vi "Open Motors.vi"(3 "error in":errorcluster, 5 "Speed PID":T8={"P"=0.04995, "I"=4.995e-05, "D"=0.4995, "F Left"=0.05, "F Right"=0.05}) -> (0 "error out":errorcluster, 1 "Right Motor Refs":T1={"DeviceStatus"={"status"=FALSE, "code"=0, "source"=""}, "Type"=enum."PWM", "PWM"={"PWM Channel"=enum."PWM 1", "DeadBand"={"Name"="", "maxPositivePwm"=0, "minPositivePwm"=0, "centerPwm"=0, "maxNegativePwm"=0, "minNegativePwm"=0, "angularRange"=0}}, "CAN"={"Device Number"=0, "Control Mode"=enum."Percent VBus", "Semaphore"=refnum, "Max Vout"=12.0, "TalonSRX Control Mode"=enum."Percent VBus"}, "Invert"=FALSE}, 2 "Left Motor Refs":T1={"DeviceStatus"={"status"=FALSE, "code"=0, "source"=""}, "Type"=enum."PWM", "PWM"={"PWM Channel"=enum."PWM 1", "DeadBand"={"Name"="", "maxPositivePwm"=0, "minPositivePwm"=0, "centerPwm"=0, "maxNegativePwm"=0, "minNegativePwm"=0, "angularRange"=0}}, "CAN"={"Device Number"=0, "Control Mode"=enum."Percent VBus", "Semaphore"=refnum, "Max Vout"=12.0, "TalonSRX Control Mode"=enum."Percent VBus"}, "Invert"=FALSE})   [LabVIEW 2015]
uses:
  <vilib>/Rock Robotics/WPI/MotorControl/WPI_MotorControlDeviceRef.ctl
  <vilib>/Rock Robotics/WPI/MotorControl/WPI_MotorControlType.ctl
  <vilib>/Rock Robotics/SystemInterfaces/DIO/FPGA_DIOPWMChannel.ctl
  <vilib>/Rock Robotics/WPI/PWM/WPI_PWMDeadband.ctl
  <vilib>/Rock Robotics/WPI/CAN/Jaguar/SubVIs/WPI_CANJaguar_ControlMode.ctl
  <vilib>/Rock Robotics/WPI/CAN/TalonSRX/WPI_CANTalonSRX_APIControlMode.ctl
  <vilib>/Rock Robotics/WPI/CAN/TalonSRX/WPI_CANTalonSRX_APIFeedbackSelect.ctl
  <vilib>/Rock Robotics/WPI/CAN/TalonSRX/WPI_CANTalonSRX_BrakeOverride.ctl
  <vilib>/Rock Robotics/WPI/MotorControl/WPI_MotorControlOpenCANTalonSRX.vi
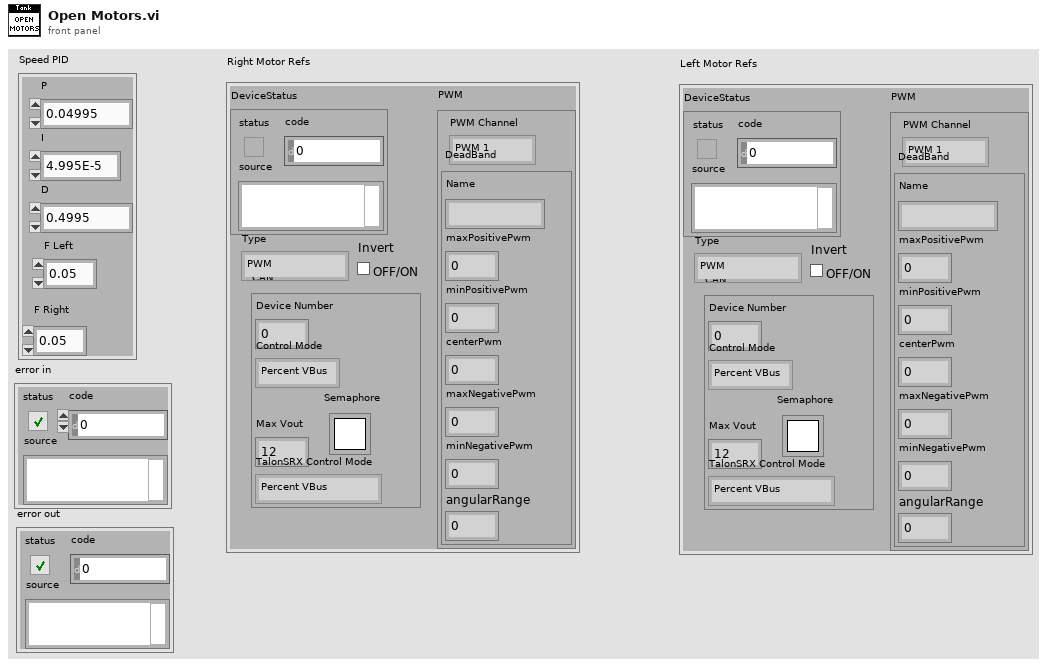
[diagram p1: front panel]
types:
  T1 = typedef "WPI_MotorControlDeviceRef.ctl" = cluster{"DeviceStatus":errorcluster, "Type":T2, "PWM":cluster{"PWM Channel":T3, "DeadBand":T4}, "CAN":cluster{"Device Number":u8, "Control Mode":T5, "Semaphore":T6, "Max Vout":dbl, "TalonSRX Control Mode":T7}, "Invert":bool}
  T2 = typedef "WPI_MotorControlType.ctl" = enum16{"PWM", "CAN", "CANTalonSRX"}
  T3 = typedef "FPGA_DIOPWMChannel.ctl" = enum8{"PWM 0", "PWM 1", "PWM 2", "PWM 3", "PWM 4", "PWM 5", "PWM 6", "PWM 7", "PWM 8", "PWM 9", "PWM MXP 0", "PWM MXP 1", "PWM MXP 2", "PWM MXP 3", "PWM MXP 4", "PWM MXP 5", "PWM MXP 6", "PWM MXP 7", "PWM MXP 8", "PWM MXP 9", "Invalid"}
  T4 = typedef "WPI_PWMDeadband.ctl" = cluster{"Name":string, "maxPositivePwm":i32, "minPositivePwm":i32, "centerPwm":i32, "maxNegativePwm":i32, "minNegativePwm":i32, "angularRange":u16}
  T5 = typedef "WPI_CANJaguar_ControlMode.ctl" = enum8{"Percent VBus", "Current", "Speed", "Position", "Voltage"}
  T6 = typedef "Semaphore RefNum" = refnum<k1>
  T7 = typedef "WPI_CANTalonSRX_APIControlMode.ctl" = enum8{"Percent VBus", "Speed", "Position", "Slave", "Unchanged / Invalid", "Voltage Compensation", "Current", "Motion Profile"}
  T8 = cluster{"P":dbl, "I":dbl, "D":dbl, "F Left":dbl, "F Right":dbl}
  T9 = typedef "WPI_CANTalonSRX_BrakeOverride.ctl" = enum8{"No Override", "Override to Coast", "Override to Brake"}
  T10 = typedef "WPI_CANTalonSRX_APIFeedbackSelect.ctl" = enum16{"Digital Quadrature Encoder", "Analog Potentiometer", "Analog Encoder", "Count on Quad-A (Rising-Edge)", "Count on Quad-A (Falling-Edge)", "CTR Magnetic Enc (Absolute)", "CTR Magnetic Enc (Relative)", "Pulse Width"}
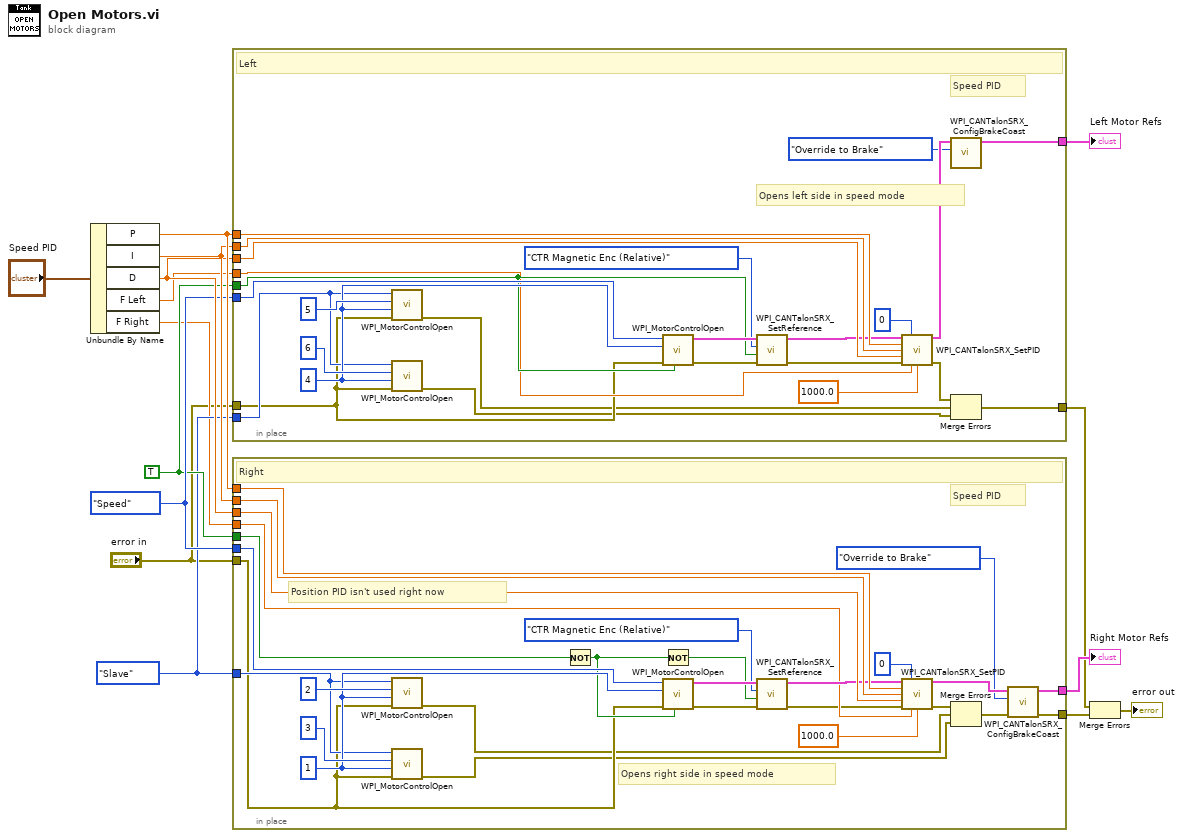
[diagram p0: block diagram]
diagram:
  w8 = TRUE ("Invert Left?")
  w7 = WPI_CANTalonSRX_APIControlMode."Slave" ("Control Mode")
  w11 = WPI_CANTalonSRX_APIControlMode."Speed" ("Control Mode")
  n1 = Unbundle By Name("Speed PID") -> ("P"=w14:dbl, "I"=w13:dbl, "D"=w12:dbl, "F Left"=w5:dbl, "F Right"=w6:dbl)
  n2 = in-place {
    in-place-border: w14 -> [w37]
    in-place-border: w13 -> [w36]
    in-place-border: w12 -> [w35]
    in-place-border: w11 -> [w34]
    in-place-border: [w17] -> w9
    in-place-border: w8 -> [w28]
    in-place-border: w7 -> [w32]
    in-place-border: w5 -> [w27]
    in-place-border: "error in" -> [w25]
    in-place-border: [w19] -> w2
    w38 = u8 4 ("Device Number")
    # "Speed PID"
    # "Opens left side in speed mode"
    # "Left"
    n3 = call-poly <vilib>:"WPI_MotorControlOpen.vi"("error in (no error)"=w25, "Master Device Number"=w38, "Device Number"=u8 5, "Control Mode"=w32) -> ("error out"=w21:errorcluster)  [unwired: 6 in, 1 out]
    n4 = call-poly <vilib>:"WPI_MotorControlOpen.vi"("error in (no error)"=w25, "Master Device Number"=w38, "Device Number"=u8 6, "Control Mode"=w32) -> ("error out"=w20:errorcluster)  [unwired: 6 in, 1 out]
    n5 = call-poly <vilib>:"WPI_MotorControlOpen.vi"("Invert"=w28, "error in (no error)"=w25, "Device Number"=w38, "Control Mode"=w34) -> ("error out"=w24:errorcluster, "MotorControlDeviceRef"=w31:T1)  [unwired: 6 in]
    n6 = call <vilib>:"WPI_CANTalonSRX_SetReference.vi"("error in (no error)"=w24, "Reverse Feedback Sensor"=w28, "Feedback Reference"=WPI_CANTalonSRX_APIFeedbackSelect."CTR Magnetic Enc (Relative)", "CAN Talon SRX Ref"=w31) -> ("error out"=w23:errorcluster, "CAN Talon SRX Ref"=w30:T1)  [unwired: 6 in]
    n7 = call <vilib>:"WPI_CANTalonSRX_SetPID.vi"("CAN Talon SRX Ref"=w30, "Parameter Slot"=u8 0, "P"=w37, "I"=w36, "D"=w35, "error in (no error)"=w23, "F"=w27, "I Zone"=1000.0) -> ("CAN Talon SRX Ref"=w18:T1, "error out"=w22:errorcluster)  [unwired: 6 in]
    n8 = call <vilib>:"WPI_CANTalonSRX_ConfigBrakeCoast.vi"("Brake / Coast Mode"=WPI_CANTalonSRX_BrakeOverride."Override to Brake", "CAN Talon SRX Ref"=w18) -> ("CAN Talon SRX Ref"=w17:T1)  [unwired: 8 in, 1 out]
    n9 = Merge Errors(w22, w21, w20) -> (w19:errorcluster)
  }
  "Left Motor Refs" <- w9
  n10 = in-place {
    in-place-border: w11 -> [w65]
    in-place-border: w14 -> [w63]
    in-place-border: w13 -> [w62]
    in-place-border: w12 -> [w61]
    in-place-border: [w44] -> w10
    in-place-border: w8 -> [w59]
    in-place-border: w7 -> [w58]
    in-place-border: w6 -> [w52]
    in-place-border: "error in" -> [w50]
    in-place-border: [w42] -> w3
    w66 = u8 1 ("Device Number")
    # "Position PID isn't used right now"
    # "Speed PID"
    # "Opens right side in speed mode"
    # "Right"
    n11 = call-poly <vilib>:"WPI_MotorControlOpen.vi"("error in (no error)"=w50, "Master Device Number"=w66, "Device Number"=u8 2, "Control Mode"=w58) -> ("error out"=w46:errorcluster)  [unwired: 6 in, 1 out]
    n12 = call-poly <vilib>:"WPI_MotorControlOpen.vi"("error in (no error)"=w50, "Master Device Number"=w66, "Device Number"=u8 3, "Control Mode"=w58) -> ("error out"=w47:errorcluster)  [unwired: 6 in, 1 out]
    n13 = Not(x=w59) -> (.not. x?=w55:bool)
    n14 = Not(x=w55) -> (.not. x?=w54:bool)
    n15 = call-poly <vilib>:"WPI_MotorControlOpen.vi"("Invert"=w55, "error in (no error)"=w50, "Device Number"=w66, "Control Mode"=w65) -> ("error out"=w49:errorcluster, "MotorControlDeviceRef"=w64:T1)  [unwired: 6 in]
    n16 = call <vilib>:"WPI_CANTalonSRX_SetReference.vi"("error in (no error)"=w49, "Reverse Feedback Sensor"=w54, "Feedback Reference"=WPI_CANTalonSRX_APIFeedbackSelect."CTR Magnetic Enc (Relative)", "CAN Talon SRX Ref"=w64) -> ("error out"=w48:errorcluster, "CAN Talon SRX Ref"=w57:T1)  [unwired: 6 in]
    n17 = call <vilib>:"WPI_CANTalonSRX_SetPID.vi"("CAN Talon SRX Ref"=w57, "Parameter Slot"=u8 0, "P"=w63, "I"=w62, "D"=w61, "error in (no error)"=w48, "F"=w52, "I Zone"=1000.0) -> ("CAN Talon SRX Ref"=w51:T1, "error out"=w45:errorcluster)  [unwired: 6 in]
    n18 = Merge Errors(w45, w46, w47) -> (w43:errorcluster)
    n19 = call <vilib>:"WPI_CANTalonSRX_ConfigBrakeCoast.vi"("error in (no error)"=w43, "Brake / Coast Mode"=WPI_CANTalonSRX_BrakeOverride."Override to Brake", "CAN Talon SRX Ref"=w51) -> ("error out"=w42:errorcluster, "CAN Talon SRX Ref"=w44:T1)  [unwired: 7 in]
  }
  "Right Motor Refs" <- w10
  n20 = Merge Errors(w2, w3) -> (→"error out":errorcluster)
